vi "Spartan HTTP Load document.vi"(7 "url path":string, 8 "error in (no error)":errorcluster, 9 "script alias":bool, 10 "File Path":path=path "c:/web", 11 "HTTP Data":T1 {"object data"."time" format="%0.2f"}) -> (0 "error out":errorcluster, 3 "Reply":T4)   [LabVIEW 2011]
uses:
  ITK EXT/http/cgi.llb/CGI Reply.ctl
  Spartan HTTP Session.ctl
  ITK EXT/http/http_obj.llb/HTTP Session Data.ctl
  ITK EXT/utils/keyedarr.llb/Keyed Array.ctl
  Summitek EXT/OpenG EXT/file/file.llb/Strip Path Extension - Path__ogtk.vi
panel:
  out "HTTP Data Out":T1 {"object data"."time" format="%0.2f"}
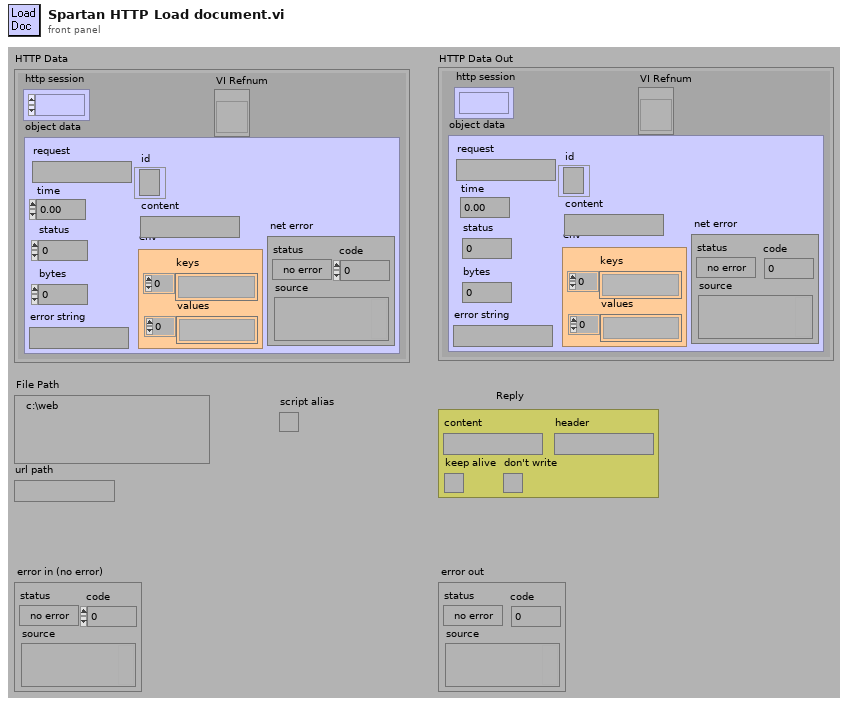
[diagram p1: front panel]
types:
  T1 = typedef "Spartan HTTP Session.ctl" = cluster{"http session":refnum<k1>, "object data":T2, "VI Refnum":refnum<vi>}
  T2 = typedef "HTTP Session Data.ctl" = cluster{"request":string, "time":dbl, "status":i32, "error string":string, "bytes":i32, "env":T3, "content":string, "id":refnum<k5>, "net error":errorcluster}
  T3 = typedef "Keyed Array.ctl" = cluster{"keys":string[], "values":string[]}
  T4 = typedef "CGI Reply.ctl" = cluster{"content":string, "header":string, "keep alive":bool, "don't write":bool}
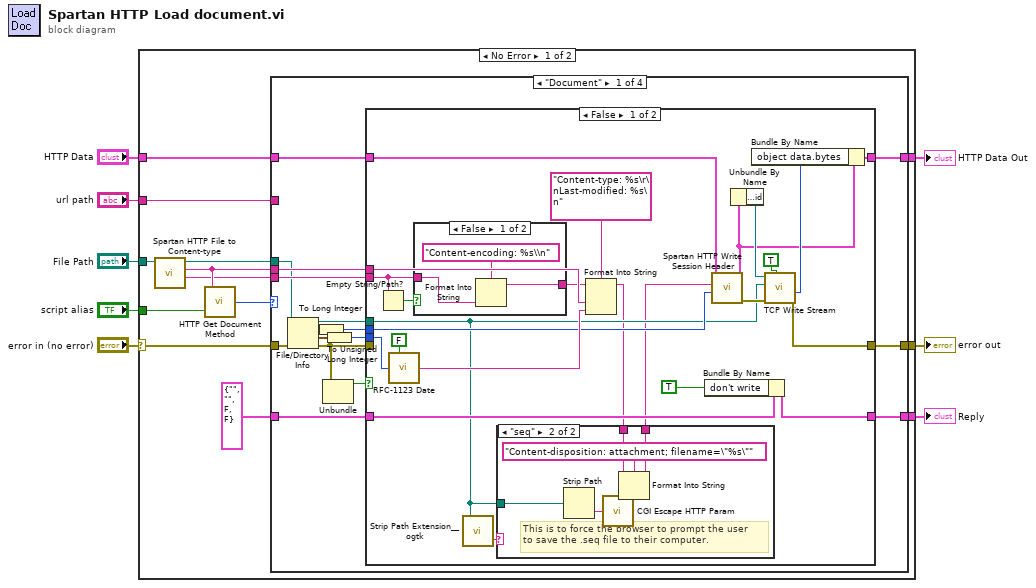
[diagram p0: block diagram]
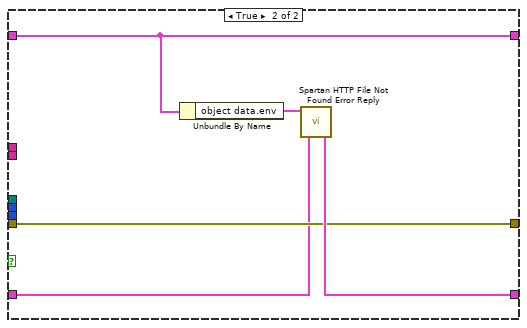
[diagram p4: hidden frame]
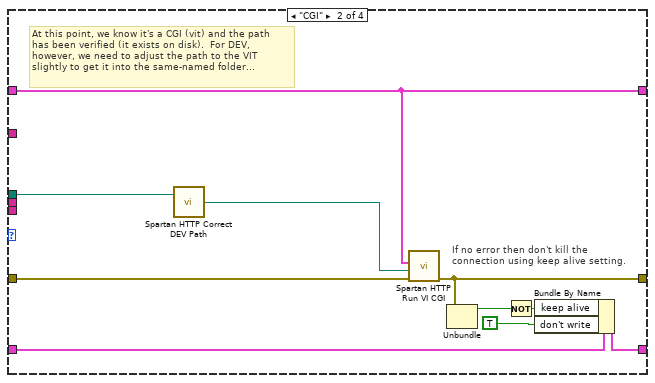
[diagram p5: hidden frame]
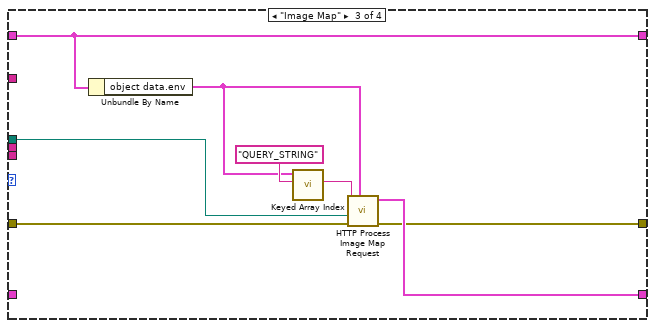
[diagram p6: hidden frame]
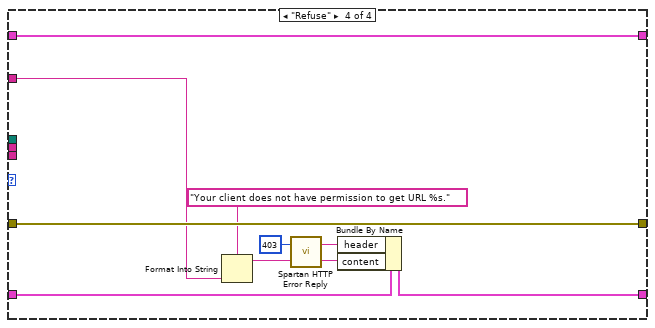
[diagram p7: hidden frame]
diagram:
  n1 = case shown="No Error" "error in (no error)" {
    selector: "error in (no error)" -> [w16 w107]
    tunnel: [w21 w107] -> w8
    tunnel: [w14 w106] -> w6
    tunnel: "HTTP Data" -> [w13 w106]
    tunnel: [w12 _] -> w4
    tunnel: "url path" -> [w11 _]
    tunnel: "File Path" -> [w10 _]
    tunnel: "script alias" -> [w9 _]
    frame No Error {
      n2 = call "Spartan HTTP File to Content-type.vi"("file path"=w10) -> ("content-encoding"=w17:string, "content-type"=w20:string, "duplicate file path"=w18:path)  [unwired: 3 in, 5 out]
      n3 = call "HTTP Get Document Method.vi"("script alias"=w9, "content-type"=w20) -> ("method"=w19:enum32{"Document", "CGI", "Image Map", "Refuse"})
      n4 = case shown="\"Document\"" w19 {
        tunnel: w20 -> [w37 _ _ _]
        tunnel: [w36 w87 w95 w99] -> w12
        tunnel: [w35 w84 w94 w105] -> w21
        tunnel: w13 -> [w34 w80 w88 w96]
        tunnel: w18 -> [w25 w79 w89 _]
        tunnel: w16 -> [w28 w86 w90 w105]
        tunnel: w17 -> [w27 _ _ _]
        tunnel: T4 {"content"="", "header"="", "keep alive"=FALSE, "don't write"=FALSE} ("Reply") -> [w24 w85 _ w98]
        tunnel: w11 -> [_ _ _ w97]
        tunnel: [w23 w80 w88 w96] -> w14
        frame "Document" {
          n5 = File/Directory Info(path=w25, error in=w28) -> (path out=w33:path, size=w22:i64, last mod=w26:timestamp, error out=w29:errorcluster)  [unwired: 3 out]
          n6 = To Long Integer(number=w22) -> (32bit integer=w32:i32)
          n7 = Unbundle(w29) -> ("status"=w30:bool)  [unwired: 2 out]
          n8 = To Unsigned Long Integer(number=w26) -> (unsigned 32bit integer=w31:u32)
          n9 = case shown="False" w30 {
            tunnel: w33 -> [w40 _]
            tunnel: [w58 w76] -> w35
            tunnel: [w57 w77] -> w36
            tunnel: w37 -> [w56 _]
            tunnel: w32 -> [w51 _]
            tunnel: w31 -> [w54 _]
            tunnel: w34 -> [w50 w73]
            tunnel: w29 -> [_ w76]
            tunnel: w27 -> [w47 _]
            tunnel: w24 -> [w44 w74]
            tunnel: [w42 w73] -> w23
            frame False {
              n10 = Empty String/Path?(string/path=w47) -> (empty?=w48:bool)
              n11 = call "RFC-1123 Date.vi"("time (now)"=w54, "numeric zone offset (true)"=FALSE) -> ("GMT Date/Time"=w53:string)
              n12 = case shown="False" w48 {
                tunnel: w47 -> [w70 w72]
                tunnel: [w69 w72] -> w46
                frame False {
                  n13 = Format Into String(format string="Content-encoding: %s\\n", w70) -> (resulting string=w69:string)  [unwired: 2 in, 1 out]
                }
                frame True {
                }
              }
              n14 = call-poly "Strip Path Extension__ogtk.vi"("path"=w40) -> ("extension"=w41:string)  [unwired: 1 out]
              n15 = Format Into String(format string="Content-type: %s\r\nLast-modified: %s\n" ("HTTP Header"), initial string=w46, w56, w53) -> (resulting string=w39:string)  [unwired: 1 in, 1 out]
              n16 = case shown="\"seq\"" w41 {
                tunnel: w39 -> [w62 w65]
                tunnel: w40 -> [_ w64]
                tunnel: [w62 w63] -> w38
                frame Default {
                }
                frame "seq" {
                  # "This is to force the browser to prompt the user\nto save the .seq file to their computer."
                  n17 = Strip Path(path=w64) -> (name=w68:string)  [unwired: 1 out]
                  n18 = call "CGI Escape HTTP Param.vi"("string"=w68) -> ("url-encoded string"=w66:string)
                  n19 = Format Into String(format string="Content-disposition: attachment; filename=\"%s\"", initial string=w65, w66) -> (resulting string=w63:string)  [unwired: 1 in, 1 out]
                }
              }
              n20 = Bundle By Name(cluster=w44, "don't write"=TRUE) -> (w57:T4)
              n21 = call "Spartan HTTP Write Session Header.vi"("content length (-1)"=w51, "header"=w38, "http session"=w50) -> ("error out"=w60:errorcluster, "http session out"=w43:T1)  [unwired: 2 in, 5 out]
              n22 = Unbundle By Name(w43) -> ("object data.id"=w49:refnum<k5>)
              n23 = call "TCP Write Stream.vi"("binary"=TRUE, "error in (no error)"=w60, "data file (<NAP>)"=w40, "connection"=w49) -> ("error out"=w58:errorcluster, "bytes written"=w45:i32)  [unwired: 2 in, 4 out]
              n24 = Bundle By Name(cluster=w43, "object data.bytes"=w45) -> (w42:T1)
            }
            frame True {
              n25 = Unbundle By Name(w73) -> ("object data.env"=w75:T3)
              n26 = call "Spartan HTTP File Not Found Error Reply.vi"("reply in"=w74, "env"=w75) -> ("reply"=w77:T4)  [unwired: 5 out]
            }
          }
        }
        frame "CGI" {
          # "At this point, we know it's a CGI (vit) and the path\nhas been verified (it exists on disk).  For DEV,\nhowever, we need to adjust the path to the VIT\nslightly to get it into the same-named folder..."
          # "If no error then don't kill the\nconnection using keep alive setting."
          n27 = call "Spartan HTTP Correct DEV Path.vi"("Normal Path"=w79) -> ("Dev Corrected Path"=w78:path)  [unwired: 4 out]
          n28 = call "Spartan HTTP Run VI CGI.vi"("error in (no error)"=w86, "cgi/vit path"=w78, "HTTP Data"=w80) -> ("error out"=w84:errorcluster)  [unwired: 3 in, 5 out]
          n29 = Unbundle(w84) -> ("status"=w82:bool)  [unwired: 2 out]
          n30 = Not(x=w82) -> (.not. x?=w81:bool)
          n31 = Bundle By Name(cluster=w85, "keep alive"=w81, "don't write"=TRUE ("keep alive")) -> (w87:T4)
        }
        frame "Image Map" {
          n32 = Unbundle By Name(w88) -> ("object data.env"=w91:T3)
          n33 = call "Keyed Array Index.vi"("key"="QUERY_STRING" ("name"), "array in"=w91) -> ("value"=w92:string)  [unwired: 2 in, 3 out]
          n34 = call "HTTP Process Image Map Request.vi"("env"=w91, "error in (no error)"=w90, "file path"=w89, "coordinates"=w92) -> ("error out"=w94:errorcluster, "Reply"=w95:T4)  [unwired: 6 out]
        }
        frame "Refuse" {
          n35 = Format Into String(format string="Your client does not have permission to get URL %s.", w97) -> (resulting string=w100:string)  [unwired: 2 in, 1 out]
          n36 = call "Spartan HTTP Error Reply.vi"("message"=w100, "status code"=403) -> ("content"=w103:string, "header"=w104:string)
          n37 = Bundle By Name(cluster=w98, "header"=w104, "content"=w103) -> (w99:T4)
        }
      }
    }
    frame Error {
    }
  }
  "error out" <- w8
  "HTTP Data Out" <- w6
  "Reply" <- w4
